vi "PH_Image.Operator.Border Control.vi"(2 "Calc GreaterBorder":dbl, 3 "Calc Smaller Border":dbl, 4 "CoG":i32, 5 "Resolution":i32) -> (0 "Greater Border":dbl, 1 "Smaller Border":dbl)   [LabVIEW 2014, in "PH_ImageOperator.lvlib"]
doc: "If \"Calc Smaller Border\" is smaller than 0 or \"Calc Greater Border\" greater than Resolution, the borders are recalculated to be symmetric relative to CoG and within 0 and Resolution."
uses:
  PH_ImageOperator.lvlib
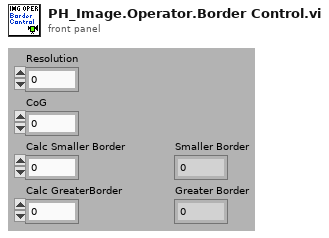
[diagram p1: front panel]
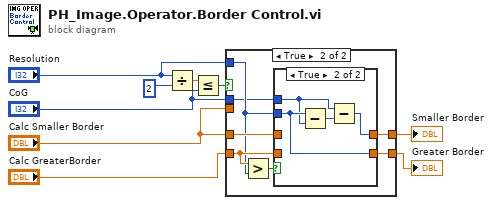
[diagram p0: block diagram]
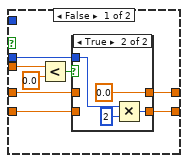
[diagram p2: hidden frame]
diagram:
  n1 = Divide(x="Resolution", y=2) -> (x/y=w3:dbl)
  n2 = Less Or Equal?(x=w3, y="CoG") -> (x <= y?=w4:bool)
  n3 = case shown="True" w4 {
    tunnel: "Calc Smaller Border" -> [w17 _]
    tunnel: [w14 w28] -> w5
    tunnel: "Calc Smaller Border" -> [w13 w29]
    tunnel: [w12 w27] -> w7
    tunnel: "Calc GreaterBorder" -> [w11 w26]
    tunnel: "CoG" -> [w10 w24]
    tunnel: "Resolution" -> [_ w25]
    frame False {
      n4 = Less?(x=w17, y=0.0) -> (x < y?=w15:bool)
      n5 = case shown="True" w15 {
        tunnel: [w19 0.0] -> w14
        tunnel: w13 -> [w19 _]
        tunnel: [w18 w22] -> w12
        tunnel: w11 -> [w18 _]
        tunnel: w10 -> [_ w20]
        frame False {
        }
        frame True {
          n6 = Multiply(x=w20, y=2) -> (x*y=w22:i32)
        }
      }
    }
    frame True {
      n7 = Greater?(x=w26, y=w25) -> (0:w30:bool)
      n8 = case shown="True" w30 {
        tunnel: w29 -> [w32 _]
        tunnel: [w32 w33] -> w28
        tunnel: [w31 w36] -> w27
        tunnel: w26 -> [w31 _]
        tunnel: w25 -> [_ w36]
        tunnel: w24 -> [_ w35]
        frame False {
        }
        frame True {
          n9 = Subtract(x=w36, y=w35) -> (x-y=w34:i32)
          n10 = Subtract(x=w35, y=w34) -> (x-y=w33:i32)
        }
      }
    }
  }
  "Greater Border" <- w7
  "Smaller Border" <- w5
